vi "Write COMPOSER Gas Mix.vi"(5 "Gas mix name":string="MyMix1", 6 "Software Version":u8, 7 "Unit ID (A)":string="A", 8 "error in":errorcluster, 9 "Gas # to store mix as":u16=236 min=236 max=255 step=1, 10 "COMPOSER gas mix input":T1={"Gas # 1"=236, "Mix % 1"=0.0, "Include # 1"=FALSE, "Gas # 2"=0, "Mix % 2"=0.0, "Include # 2"=FALSE, "Gas # 3"=0, "Mix % 3"=0.0, "Include # 3"=FALSE, "Gas # 4"=0, "Mix % 4"=0.0, "Include # 4"=FALSE, "Gas # 5"=0, "Mix % 5"=0.0, "Include # 5"=FALSE} {"Gas # 1" max=255 step=1; "Mix % 1" min=0.0 max=100.0 step=0.01; "Gas # 2" max=255 step=1; "Mix % 2" min=0.0 max=100.0 step=0.01; "Gas # 3" max=255 step=1; "Mix % 3" min=0.0 max=100.0 step=0.01; "Gas # 4" max=255 step=1; "Mix % 4" min=0.0 max=100.0 step=0.01; "Gas # 5" max=255 step=1; "Mix % 5" min=0.0 max=100.0 step=0.01}, 11 "VISA Session In":refnum<visa-resource-name>="Alicat") -> (0 "error out":errorcluster, 2 "Completion text":string, 3 "VISA Session Out":refnum<visa-resource-name>)   [LabVIEW 2020]
doc: "Writes a new COMPOSER gas mix with the specified gas concentrations, gas name (up to 6 characters), and gas number (236-255).\n\nThis can be used to update a currently selected COMPOSER gas mix in real time."
uses:
  <vilib>/Instr/_visa.llb/VISA Flush IO Buffer Mask.ctl
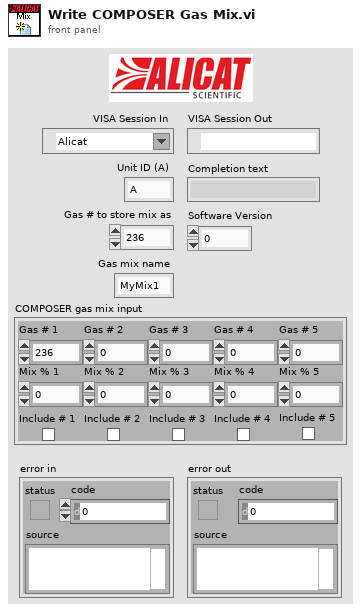
[diagram p1: front panel]
types:
  T1 = cluster{"Gas # 1":u16, "Mix % 1":dbl, "Include # 1":bool, "Gas # 2":u16, "Mix % 2":dbl, "Include # 2":bool, "Gas # 3":u16, "Mix % 3":dbl, "Include # 3":bool, "Gas # 4":u16, "Mix % 4":dbl, "Include # 4":bool, "Gas # 5":u16, "Mix % 5":dbl, "Include # 5":bool}
  T2 = typedef "VISA Flush IO Buffer Mask.ctl" = u16
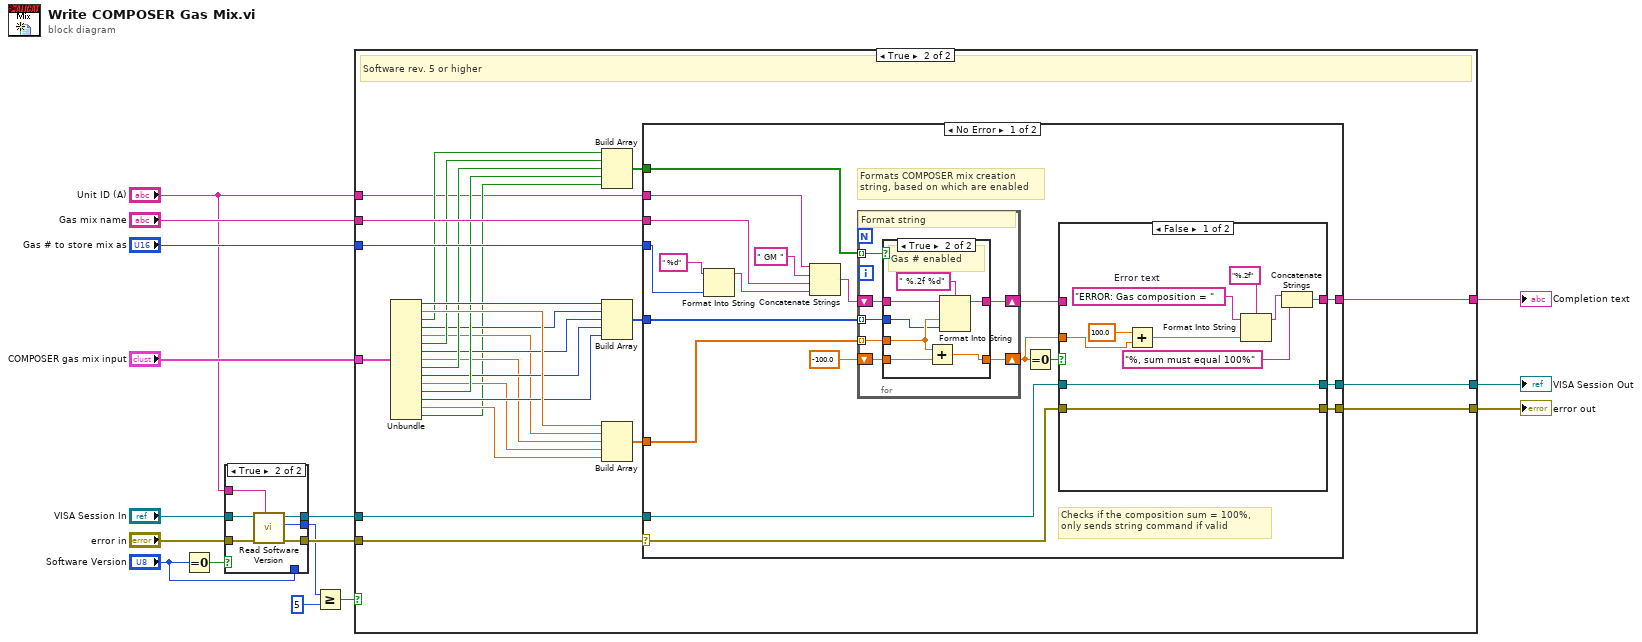
[diagram p0: block diagram]
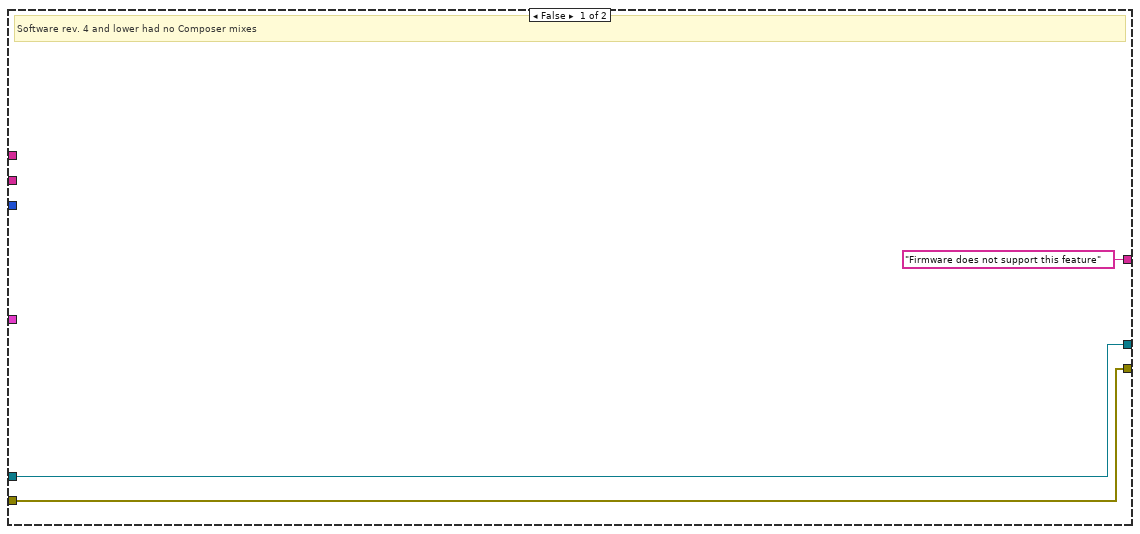
[diagram p2: hidden frame]
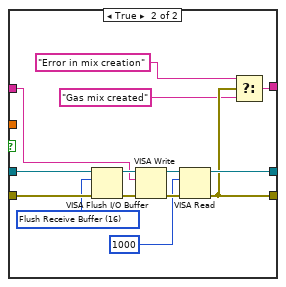
[diagram p3: hidden frame]
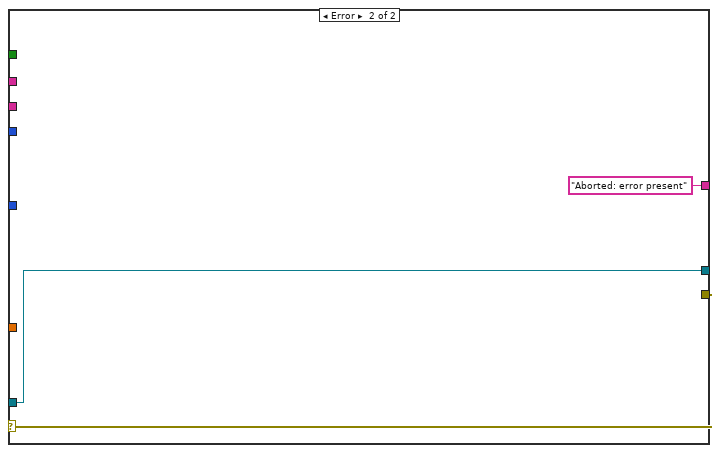
[diagram p5: hidden frame]
diagram:
  n1 = Equal To 0?(x="Software Version") -> (x = 0?=w11:bool)
  n2 = case shown="True" w11 {
    tunnel: "error in" -> [w18 w25]
    tunnel: "VISA Session In" -> [w17 w24]
    tunnel: "Unit ID (A)" -> [_ w23]
    tunnel: [w18 w22] -> w8
    tunnel: [w17 w21] -> w9
    tunnel: [w19 w20] -> w3
    tunnel: "Software Version" -> [w19 _]
    frame False {
    }
    frame True {
      n3 = call "Read Software Version.vi"("Unit ID (A)"=w23, "error in"=w25, "VISA Session In"=w24) -> ("error out"=w22:errorcluster, "Software Version"=w20:u8, "VISA Session Out"=w21:refnum<visa-resource-name>)  [unwired: 6 in]
    }
  }
  n4 = Greater Or Equal?(x=w3, y=u8 5) -> (x >= y?=w1:bool)
  n5 = case shown="True" w1 {
    tunnel: [w27 w55] -> w16
    tunnel: [w26 w54] -> w15
    tunnel: "Gas mix name" -> [_ w51]
    tunnel: "Gas # to store mix as" -> [_ w50]
    tunnel: "COMPOSER gas mix input" -> [_ w48]
    tunnel: w9 -> [w27 w32]
    tunnel: w8 -> [w26 w31]
    tunnel: "Unit ID (A)" -> [_ w30]
    tunnel: ["Firmware does not support this feature" ("Completion text") w29] -> w2
    frame False {
      # "Software rev. 4 and lower had no Composer mixes"
    }
    frame True {
      # "Software rev. 5 or higher"
      n6 = Unbundle(w48) -> ("Gas # 1"=w47:u16, "Mix % 1"=w46:dbl, "Include # 1"=w45:bool, "Gas # 2"=w41:u16, "Mix % 2"=w37:dbl, "Include # 2"=w44:bool, "Gas # 3"=w40:u16, "Mix % 3"=w36:dbl, "Include # 3"=w43:bool, "Gas # 4"=w39:u16, "Mix % 4"=w35:dbl, "Include # 4"=w42:bool, "Gas # 5"=w38:u16, "Mix % 5"=w34:dbl, "Include # 5"=w33:bool)
      n7 = Build Array(w45, w44, w43, w42, w33) -> (w49:bool[])
      n8 = Build Array(w47, w41, w40, w39, w38) -> (w53:u16[])
      n9 = Build Array(w46, w37, w36, w35, w34) -> (w52:dbl[])
      n10 = case shown="No Error" w31 {
        selector: w31 -> [w59 w116]
        tunnel: w32 -> [w74 w117]
        tunnel: [w73 w117] -> w55
        tunnel: [w72 w116] -> w54
        tunnel: w53 -> [w71 _]
        tunnel: w52 -> [w70 _]
        tunnel: w30 -> [w69 _]
        tunnel: w51 -> [w67 _]
        tunnel: w50 -> [w65 _]
        tunnel: w49 -> [w58 _]
        tunnel: [w56 "Aborted: error present" ("Completion text")] -> w29
        frame No Error {
          # "Checks if the composition sum = 100%,\nonly sends string command if valid"
          # "Formats COMPOSER mix creation\nstring, based on which are enabled"
          n11 = Format Into String(format string=" %d", w65) -> (resulting string=w63:string)  [unwired: 2 in, 1 out]
          n12 = Concatenate Strings(w69, " GM " ("resulting string"), w67, w63) -> (w66:string)
          n13 = for {
            tunnel: w71 -> [w105] mode=indexing
            tunnel: w70 -> [w101] mode=indexing
            shift-right: [w104] -> w60
            shift-left: w66 -> [w103]
            shift-right: [w100] -> w57
            shift-left: -100.0 ("Composition % 5") -> [w102]
            tunnel: w58 -> [w99] mode=indexing
            # "Format string"
            n14 = case shown="True" w99 {
              tunnel: w105 -> [_ w108]
              tunnel: [w106 w113] -> w104
              tunnel: w103 -> [w106 w112]
              tunnel: w102 -> [w107 w111]
              tunnel: w101 -> [_ w109]
              tunnel: [w107 w110] -> w100
              frame False {
                # "Disabled"
              }
              frame True {
                # "Gas # enabled"
                n15 = Add(x=w109, y=w111) -> (x+y=w110:dbl)
                n16 = Format Into String(format string=" %.2f %d", initial string=w112, w109, w108) -> (resulting string=w113:string)  [unwired: 1 in, 1 out]
              }
            }
          }
          n17 = Equal To 0?(x=w57) -> (x = 0?=w61:bool)
          n18 = case shown="False" w61 {
            tunnel: w74 -> [w83 w98]
            tunnel: [w83 w97] -> w73
            tunnel: [w84 w87] -> w72
            tunnel: w59 -> [w84 w96]
            tunnel: [w80 w88] -> w56
            tunnel: w60 -> [_ w89]
            tunnel: w57 -> [w75 _]
            frame False {
              w82 = "ERROR: Gas composition = "  # Error text
              n19 = Add(x=100.0, y=w75) -> (x+y=w76:dbl)
              n20 = Format Into String(format string="%.2f", initial string=w82, w76) -> (resulting string=w79:string)  [unwired: 1 in, 1 out]
              n21 = Concatenate Strings(w79, "%, sum must equal 100%" ("string")) -> (w80:string)
            }
            frame True {
              w91 = T2 16 items=["Flush Receive Buffer"=16, "Write Transmit Buffer to Device"=32, "Flush Receive Buffer (No I/O)"=64, "Flush Transmit Buffer"=128] ("Mask")
              n22 = VISA Flush I/O Buffer(VISA resource name=w98, mask (16)=w91, error in (no error)=w96) -> (VISA resource name out=w94:refnum<visa-resource-name>, error out=w90:errorcluster)
              n23 = VISA Write(VISA resource name=w94, write buffer=w89, error in (no error)=w90) -> (VISA resource name out=w93:refnum<visa-resource-name>, error out=w95:errorcluster)  [unwired: 1 out]
              n24 = VISA Read(VISA resource name=w93, byte count=u32 1000, error in (no error)=w95) -> (VISA resource name out=w97:refnum<visa-resource-name>, error out=w87:errorcluster)  [unwired: 2 out]
              n25 = Select(t="Error in mix creation" ("Completion text"), s=w87, f="Gas mix created") -> (s? t:f=w88:string)
            }
          }
        }
        frame Error {
        }
      }
    }
  }
  "error out" <- w15
  "VISA Session Out" <- w16
  "Completion text" <- w2
